vi "Prepare Error Template.vi"(8 "error in (no error)":errorcluster, 10 "error":T1, 11 "templates directory":path) -> (0 "error out":errorcluster)   [LabVIEW 2016]
uses:
  Error File Management/Controls/NI Error.ctl
  <vilib>/Utility/miscctls.llb/LVDeltaXY32Cluster.ctl
  <vilib>/Utility/traverseref.llb/TRef TravTarget.ctl
  <vilib>/Utility/traverseref.llb/VI Scripting - Traverse.lvlib
  Error File Management/Error File Management.lvlib
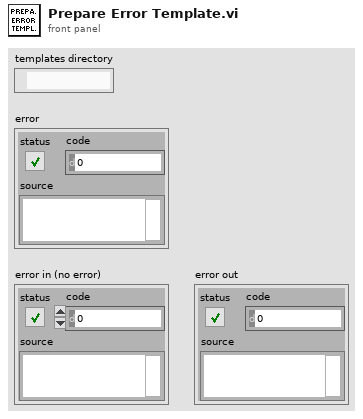
[diagram p1: front panel]
types:
  T1 = typedef "Error File Management.lvlib/NI Error.ctl" = errorcluster
  T2 = typedef "LVDeltaXY32Cluster.ctl" = cluster{"X":i32, "Y":i32}
  T3 = typedef "TRef TravTarget.ctl" = enum16{"FP", "BD", "Other"}
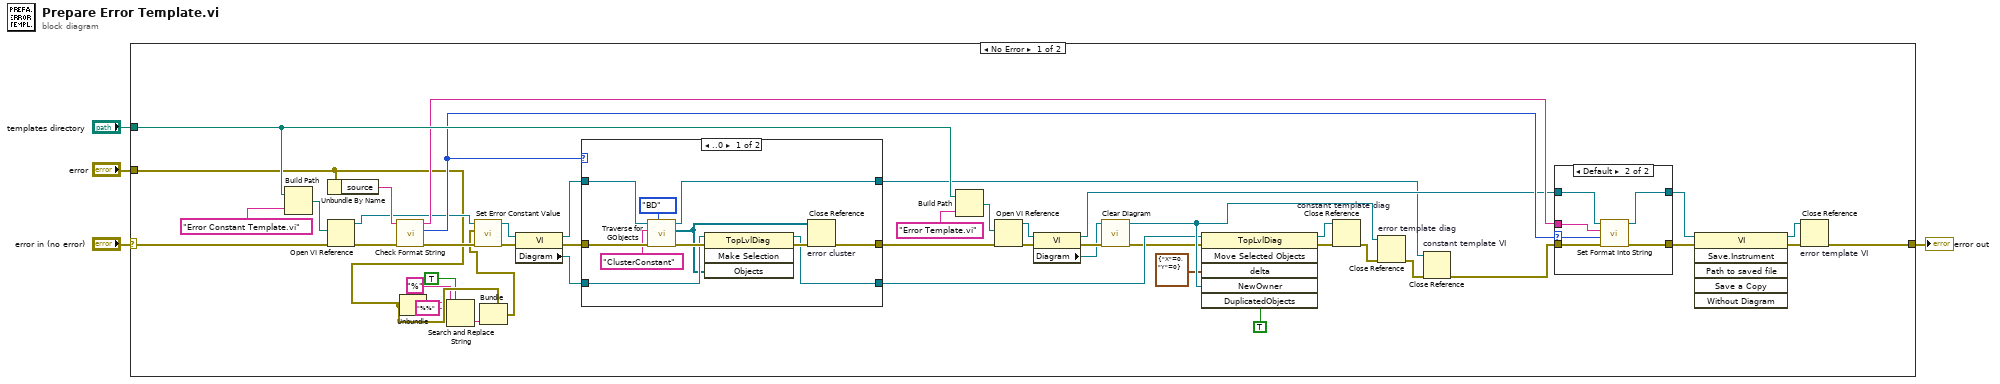
[diagram p0: block diagram]
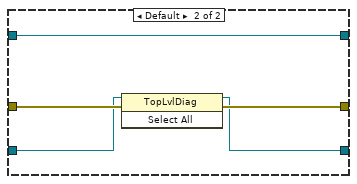
[diagram p2: hidden frame]
diagram:
  n1 = case shown="No Error" "error in (no error)" {
    selector: "error in (no error)" -> [w12 w75]
    tunnel: "error" -> [w11 _]
    tunnel: "templates directory" -> [w47 _]
    tunnel: [w17 w75] -> w2
    frame No Error {
      n2 = Build Path(base path=w47, name or relative path="Error Constant Template.vi") -> (appended path=w42:path)
      n3 = Unbundle By Name(w11) -> ("source"=w45:string)
      n4 = Open VI Reference(vi path=w42, error in (no error)=w12) -> (vi reference=w19:refnum<vi>, error out=w43:errorcluster)  [unwired: 4 in]
      n5 = call "Check Format String.vi"("error in (no error)"=w43, "format string in"=w45) -> ("error out"=w44:errorcluster, "# of format strings"=w38:i32, "format string out"=w37:string)  [unwired: 7 in]
      n6 = Unbundle(w11) -> ("source"=w10:string)  [unwired: 2 out]
      n7 = Search and Replace String(replace all?=TRUE ("replace all? (F)"), input string=w10, search string="%%", replace string="%" ("replace string (\"\")")) -> (result string=w9:string)  [unwired: 4 in, 3 out]
      n8 = Bundle(cluster=w11, "source"=w9) -> (w8:T1)  [unwired: 2 in]
      n9 = call "Set Error Constant Value.vi"("error in (no error)"=w44, "error"=w8, "VI in"=w19) -> ("error out"=w20:errorcluster, "VI out"=w30:refnum<vi>)  [unwired: 7 in]
      n10 = property class="VI"(reference=w30, error in=w20) -> (reference out=w32:refnum<vi>, error out=w15:errorcluster, "Diagram"=w27:refnum<vi>)
      n11 = case shown="..0" w38 {
        tunnel: [w58 w63] -> w24
        tunnel: w27 -> [w57 w64]
        tunnel: [w52 w66] -> w46
        tunnel: w15 -> [w60 w65]
        tunnel: w32 -> [w54 w62]
        tunnel: [w53 w62] -> w33
        frame ..0 {
          n12 = call <vilib>:"Traverse for GObjects.vi"("Traverse Target"=TRef_TravTarget."BD", "error in (no error)"=w60, "Class Name"="ClusterConstant", "VI Refnum"=w54) -> ("error out"=w59:errorcluster, "References"=w51:refnum<vi>[], "dup VI Refnum"=w53:refnum<vi>)  [unwired: 4 in, 1 out]
          n13 = invoke class="TopLvlDiag" method="Make Selection"(reference=w57, error in=w59, "Objects"=w51) -> (reference out=w58:refnum<vi>, error out=w61:errorcluster)  [unwired: 1 in, 2 out]
          n14 = Close Reference "error cluster"(reference=w51, error in (no error)=w61) -> (error out=w52:errorcluster)
        }
        frame Default {
          n15 = invoke class="TopLvlDiag" method="Select All"(reference=w64, error in=w65) -> (reference out=w63:refnum<vi>, error out=w66:errorcluster)  [unwired: 1 in, 1 out]
        }
      }
      n16 = Build Path(base path=w47, name or relative path="Error Template.vi") -> (appended path=w40:path)
      n17 = Open VI Reference(vi path=w40, error in (no error)=w46) -> (vi reference=w21:refnum<vi>, error out=w22:errorcluster)  [unwired: 4 in]
      n18 = property class="VI"(reference=w21, error in=w22) -> (reference out=w34:refnum<vi>, error out=w50:errorcluster, "Diagram"=w23:refnum<vi>)
      n19 = call "Clear Diagram.vi"("error in (no error)"=w50, "top lvl diag in"=w23) -> ("error out"=w13:errorcluster, "top lvl diag out"=w49:refnum<vi>)  [unwired: 8 in]
      n20 = invoke class="TopLvlDiag" method="Move Selected Objects"(reference=w24, error in=w13, "delta"=T2 {"X"=0, "Y"=0} ("X/Y Delta"), "NewOwner"=w49, "DuplicatedObjects"=TRUE ("Duplicate?")) -> (reference out=w28:refnum<vi>, error out=w29:errorcluster)  [unwired: 1 in, 4 out]
      n21 = Close Reference "constant template diag"(reference=w28, error in (no error)=w29) -> (error out=w31:errorcluster)
      n22 = Close Reference "error template diag"(reference=w49, error in (no error)=w31) -> (error out=w48:errorcluster)
      n23 = Close Reference "constant template VI"(reference=w33, error in (no error)=w48) -> (error out=w14:errorcluster)
      n24 = case shown="Default" w38 {
        selector: w38 -> [_ w69]
        tunnel: w14 -> [w68 w74]
        tunnel: w34 -> [w67 w73]
        tunnel: [w67 w72] -> w35
        tunnel: [w68 w71] -> w36
        tunnel: w37 -> [_ w70]
        frame ..0 {
        }
        frame Default {
          n25 = call "Set Format Into String.vi"("error in (no error)"=w74, "# of format strings (0)"=w69, "format string"=w70, "VI in"=w73) -> ("error out"=w71:errorcluster, "VI out"=w72:refnum<vi>)  [unwired: 6 in]
        }
      }
      n26 = invoke class="VI" method="Save.Instrument"(reference=w35, error in=w36) -> (reference out=w18:refnum<vi>, error out=w16:errorcluster)  [unwired: 4 in, 4 out]
      n27 = Close Reference "error template VI"(reference=w18, error in (no error)=w16) -> (error out=w17:errorcluster)
    }
    frame Error {
    }
  }
  "error out" <- w2
